vi "Show Display Settings Dialog.vi"(8 "error in (no error)":errorcluster, 11 "IMAQ Display in":refnum<class "HIJ Vision Display.lvclass">) -> (0 "error out":errorcluster, 3 "IMAQ Display out":refnum<class "HIJ Vision Display.lvclass">)   [LabVIEW 2014, in "HIJ Vision Display.lvlib" / "HIJ Vision Display.lvclass"]
uses:
  HIJ Vision Display.lvclass
  Display Settings Dialog/Display Settings Dialog/Display Settings Dialog.lvclass
  HIJ Vision Display.lvclass/HIJ Vision Display.ctl
  Display Settings Dialog/Display Settings Dialog/Display Settings Dialog.lvclass/Display Settings Dialog.ctl
  <vilib>/ActorFramework/Actor/Actor.lvclass
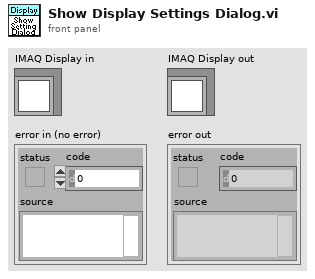
[diagram p1: front panel]
types:
  T1 = typedef "HIJ Vision Display.lvlib/HIJ Vision Display.lvclass/DisplaySettings.ctl" = cluster{"Min. Thresh.":sgl, "X":dbl, "Y":dbl, "ShowLineout":bool, "ScaleParts":i32, "ShowLegende":bool, "Target Cross":bool, "Centroid Cross":bool, "Target color":u32, "Centroid color":u32, "calibr. µm/px":sgl[unit]}
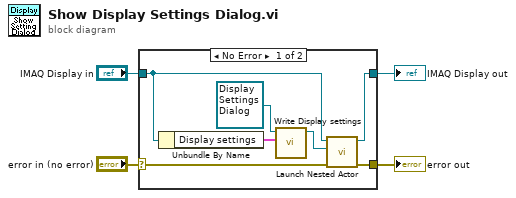
[diagram p0: block diagram]
diagram:
  n1 = case shown="No Error" "error in (no error)" {
    selector: "error in (no error)" -> [w10 w13]
    tunnel: [w9 w13] -> w3
    tunnel: [w11 w12] -> w1
    tunnel: "IMAQ Display in" -> [w7 w12]
    frame No Error {
      n2 = Unbundle By Name(w7) -> ("Display settings"=w5:T1)
      n3 = call "Write Display settings.vi"("Display settings"=w5, "Display Settings Dialog in"=refnum<class "Display Settings Dialog.lvclass"> refnum ("Display Settings Dialog.lvlib:Display Settings Dialog.lvclass")) -> ("Display Settings Dialog out"=w6:refnum<class "Display Settings Dialog.lvclass">)  [unwired: 8 in, 1 out]
      n4 = call <vilib>:"Launch Nested Actor.vi"("error in (no error)"=w10, "Nested Actor"=w6, "Caller Actor in"=w7) -> ("error out"=w9:errorcluster, "Caller Actor out"=w11:refnum<class "HIJ Vision Display.lvclass">)  [unwired: 6 in, 1 out]
    }
    frame Error {
    }
  }
  "error out" <- w3
  "IMAQ Display out" <- w1
